vi "Read Send Text Data.vi"(8 "error in (no error)":errorcluster, 9 "number of registers":u16, 10 "starting address":u16, 11 "device data model in":refnum<class "WebSocket Data Model.lvclass">) -> (0 "error out":errorcluster, 2 "data":string, 3 "device data model out":refnum<class "WebSocket Data Model.lvclass">)   [LabVIEW 2021, in "WebSockets.lvlib" / "WebSocket Data Model.lvclass"]
doc: "Reads N input registers from the device model, starting at register M."
uses:
  WebSocket Data Model.lvclass
  WebSocket Data Model.lvclass/WebSocket Data Model.ctl
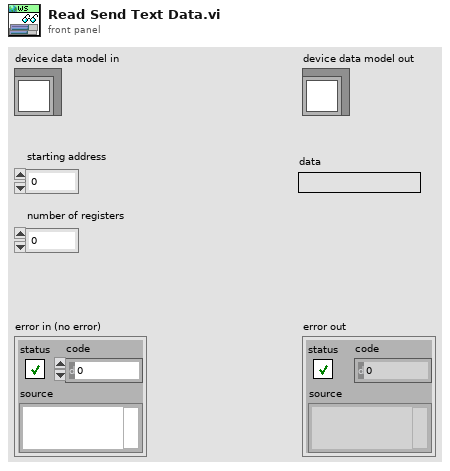
[diagram p1: front panel]
types:
  T1 = typedef "WebSockets.lvlib/WebSocket Data Model.lvclass/Data Model.ctl" = cluster{"UTC":u64, "Receive Binary Data":u8[], "Receive Text Data":string, "Send Binary Data":u8[], "Send Text Data":string, "ES":u8}
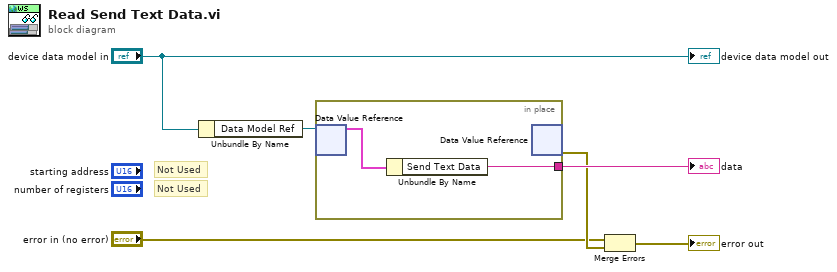
[diagram p0: block diagram]
diagram:
  # "Not Used"
  # "Not Used"
  n1 = Unbundle By Name("device data model in") -> ("Data Model Ref"=w3:refnum<data-value>)
  n2 = in-place {
    in-place-border: [w7] -> w5
    n3 = in-place-dvr #1(w3) -> (w8:T1)  [unwired: 1 out]
    n4 = Unbundle By Name(w8) -> ("Send Text Data"=w7:string)
    n5 = in-place-dvr #1() -> (w2:errorcluster)  [unwired: 1 in, 1 out]
  }
  "data" <- w5
  n6 = Merge Errors("error in (no error)", w2) -> (→"error out":errorcluster)
  "device data model out" <- "device data model in"
